vi "EvaluatePoint_v2.vi"(0 "object in":refnum<class "Evaluator.lvclass">, 2 "Game":refnum<class "Game.lvclass">, 3 "point":dbl[](array[numeric]), 5 "error in (no error)":errorcluster) -> (14 "object out":refnum<class "Evaluator.lvclass">, 19 "error out":errorcluster)   [LabVIEW 2023, in "Evaluator.lvclass"]
uses:
  Evaluator.lvclass
  Game_class/Game.lvclass
  Evaluator.lvclass/Evaluator.ctl
  Game_class/Game.lvclass/Game.ctl
  Game_class/Read Utilities.lvclass.vi
  Game_class/Write Utilities.lvclass.vi
  Utilities_class/Utilities.lvclass
panel:
  out "evaluation":dbl
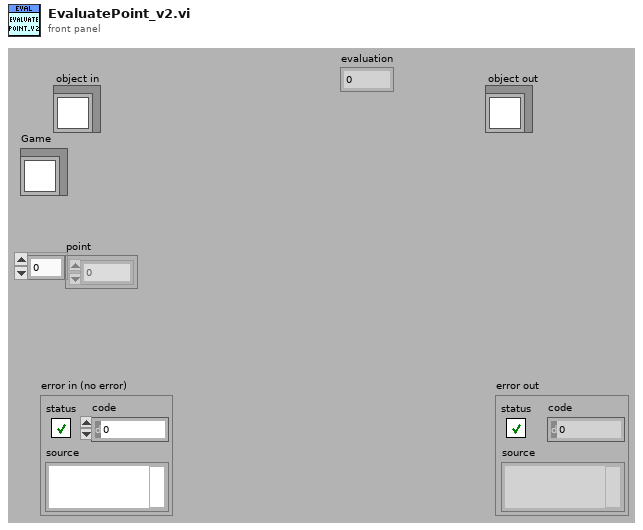
[diagram p1: front panel]
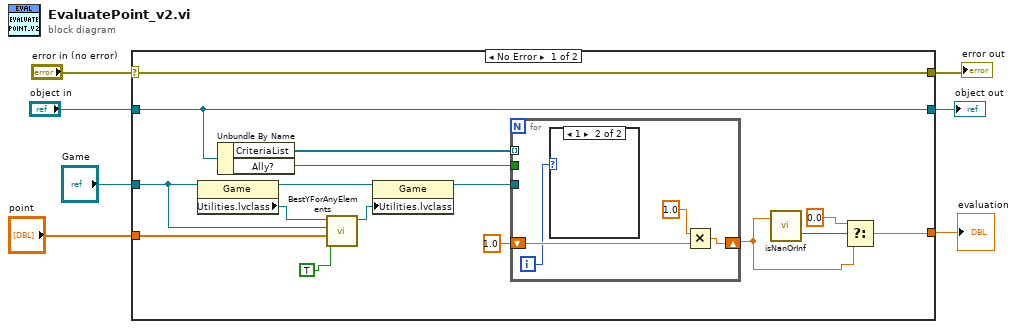
[diagram p0: block diagram]
diagram:
  n1 = case shown="No Error" "error in (no error)" {
    selector: "error in (no error)" -> [w23 w29]
    tunnel: [w23 w29] -> w6
    tunnel: [w22 w28] -> w4
    tunnel: "object in" -> [w22 w28]
    tunnel: "Game" -> [w11 _]
    tunnel: "point" -> [w9 _]
    tunnel: [w8 _] -> w1
    frame No Error {
      n2 = property class="Game"(reference=w11) -> (reference out=w12:refnum<class "Game.lvclass">, "Utilities.lvclass"=w15:refnum<class "Utilities.lvclass">)  [unwired: 1 in, 1 out]
      n3 = Unbundle By Name(w22) -> ("CriteriaList"=w17:refnum<class "Criterion.lvclass">[], "Ally?"=w16:bool)
      n4 = call "BestYForAnyElements.vi"("inimigos"=TRUE, "Position to be analyzed"=w9, "Game"=w11, "Utilities in"=w15) -> ("Utilities out"=w13:refnum<class "Utilities.lvclass">)  [unwired: 4 in, 3 out]
      n5 = property class="Game"(reference=w12, "Utilities.lvclass"=w13) -> (reference out=w10:refnum<class "Game.lvclass">)  [unwired: 1 in, 1 out]
      n6 = for {
        shift-right: [w26] -> w18
        shift-left: 1.0 -> [w27]
        tunnel: w17 -> [_] mode=indexing
        tunnel: w16 -> [_]
        tunnel: w10 -> [_]
        i -> [w25]
        n7 = case shown="1" w25 {
          frame 0, Default {
          }
          frame 1 {
          }
        }
        n8 = Multiply(x=1.0, y=w27) -> (x*y=w26:dbl)
      }
      n9 = call "isNanOrInf.vi"("value"=w18) -> ("narOrInf?"=w20:bool)  [unwired: 13 in, 5 out]
      n10 = Select(t=0.0, s=w20, f=w18) -> (s? t:f=w8:dbl)
    }
    frame Error {
    }
  }
  "error out" <- w6
  "object out" <- w4
  "evaluation" <- w1
